vi "ProgG_003_MG.vi"() -> ()   [LabVIEW 2021]
panel:
  out "Wynik":ext=5.5500000000000000002
  in  "y":ext=2.22
  in  "x":ext=7.77
  in  "?":bool
  # "x+y"
  # "x-y"
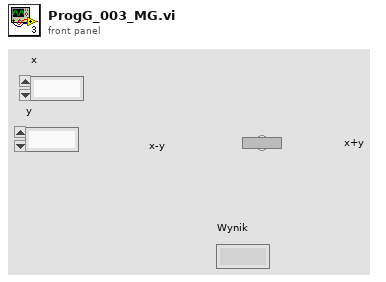
[diagram p1: front panel]
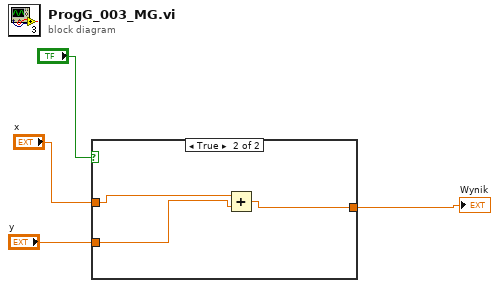
[diagram p0: block diagram]
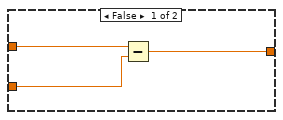
[diagram p2: hidden frame]
diagram:
  n1 = case shown="True" "?" {
    tunnel: "x" -> [w7 w10]
    tunnel: "y" -> [w6 w9]
    tunnel: [w5 w8] -> w2
    frame False {
      n2 = Subtract(x=w7, y=w6) -> (x-y=w5:ext)
    }
    frame True {
      n3 = Add(x=w10, y=w9) -> (x+y=w8:ext)
    }
  }
  "Wynik" <- w2
